vi "Generate INSERT SQL Query for Temporary Table.vi"(8 "error in (no error)":errorcluster, 11 "Importing Transactions":refnum<class "TransactionList.lvclass">) -> (0 "error out":errorcluster, 2 "INSERT Query":string, 3 "Statement.lvclass":refnum<class "TransactionList.lvclass">)   [LabVIEW 2018, in "TransactionList.lvclass"]
uses:
  TransactionList.lvclass
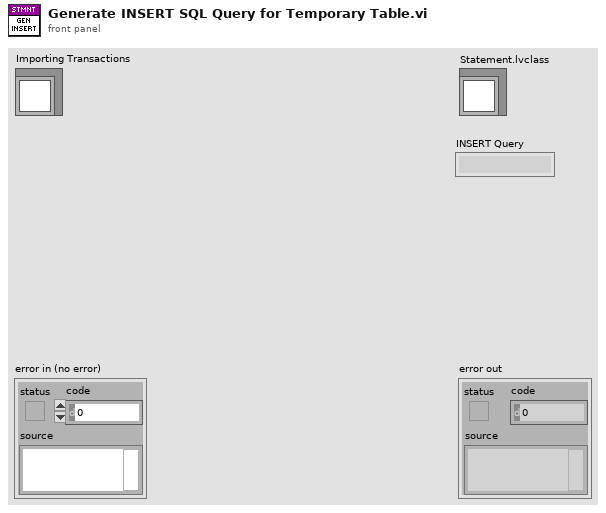
[diagram p1: front panel]
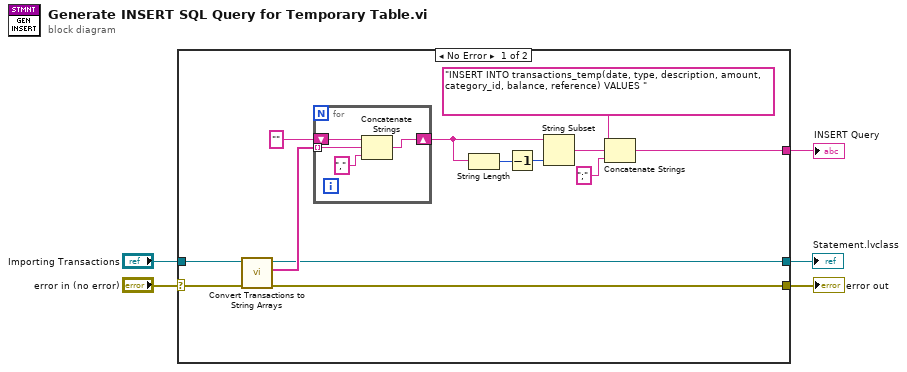
[diagram p0: block diagram]
diagram:
  n1 = case shown="No Error" "error in (no error)" {
    selector: "error in (no error)" -> [w9 w24]
    tunnel: [w8 w24] -> w4
    tunnel: "Importing Transactions" -> [w10 w23]
    tunnel: [w13 _] -> w2
    tunnel: [w6 w23] -> w1
    frame No Error {
      n2 = call-dynamic "Convert Transactions to String Arrays.vi"("error in (no error)"=w9, "Statement in"=w10) -> ("error out"=w8:errorcluster, "String Arrays"=w7:string[], "Statement out"=w6:refnum<class "TransactionList.lvclass">)  [unwired: 7 in]
      n3 = for {
        shift-right: [w22] -> w11
        shift-left: "" -> [w21]
        tunnel: w7 -> [w19] mode=indexing
        n4 = Concatenate Strings(w21, w19, "," ("string")) -> (w22:string)
      }
      n5 = String Length(string=w11) -> (length=w15:i32)
      n6 = Decrement(x=w15) -> (x-1=w16:i32)
      n7 = String Subset(string=w11, length (rest)=w16) -> (substring=w17:string)  [unwired: 1 in]
      n8 = Concatenate Strings("INSERT INTO transactions_temp(date, type, description, amount, category_id, balance, reference) VALUES ", w17, ";" ("string")) -> (w13:string)
    }
    frame Error {
    }
  }
  "error out" <- w4
  "INSERT Query" <- w2
  "Statement.lvclass" <- w1
